vi "PiezoZeroAxis.vi"(8 "error in (no error)":errorcluster, 11 "reference":refnum<k7>) -> (0 "error out":errorcluster, 3 "reference out":refnum<k7>)   [LabVIEW 2018]
uses:
  <userlib>/bpc203/PiezoChannelNumber.ctl
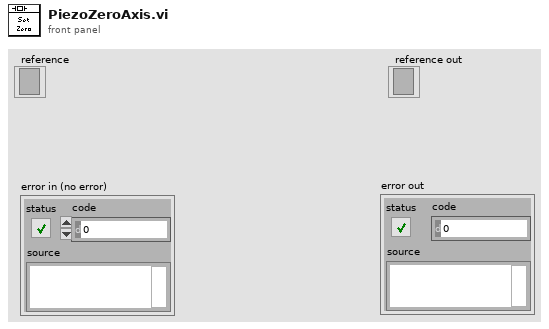
[diagram p1: front panel]
types:
  T1 = typedef "PiezoChannelNumber.ctl" = u16
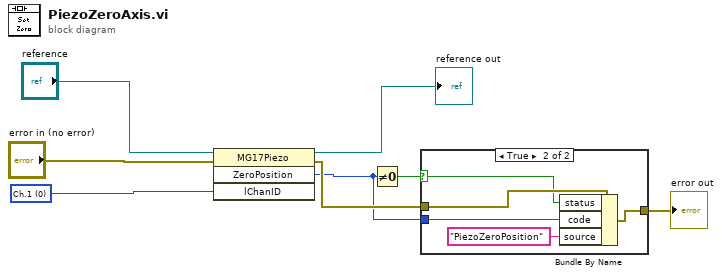
[diagram p0: block diagram]
diagram:
  w6 = T1 0 items=["Ch.1", "Ch.2"] ("lChanID")
  n1 = invoke class="MG17Piezo" method="ZeroPosition"(reference="reference", error in="error in (no error)", "lChanID"=w6) -> (reference out=→"reference out":refnum<k7>, error out=w3:errorcluster, "ZeroPosition"=w1:i32)  [unwired: 1 in, 1 out]
  n2 = Not Equal To 0?(x=w1) -> (x != 0?=w4:bool)
  n3 = case shown="True" w4 {
    selector: w4 -> [_ w13]
    tunnel: w3 -> [w9 w14]
    tunnel: [w9 w11] -> w2
    tunnel: w1 -> [_ w10]
    frame False {
    }
    frame True {
      n4 = Bundle By Name(cluster=w14, "status"=w13, "code"=w10, "source"="PiezoZeroPosition") -> (w11:errorcluster)
    }
  }
  "error out" <- w2
